vi "isVerbose.vi"(11 "Test Assert in":refnum<class "Test Assert.lvclass">) -> (2 "Verbose":bool, 3 "Test Assert out":refnum<class "Test Assert.lvclass">)   [LabVIEW 2013, in "Caraya.lvlib" / "Test Assert.lvclass"]
uses:
  Test Assert.lvclass
  Test Assert.lvclass/Test Assert.ctl
  Test Manager/Test Manager.lvclass/Test Manager.ctl
  Test Manager/Test Manager.lvclass
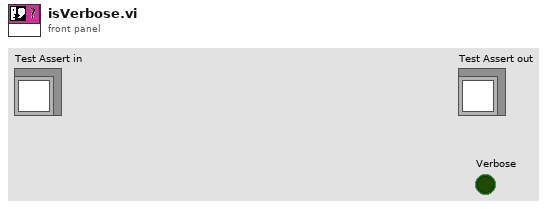
[diagram p1: front panel]
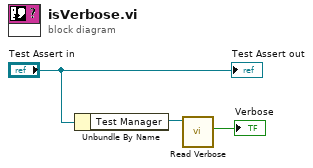
[diagram p0: block diagram]
diagram:
  n1 = Unbundle By Name("Test Assert in") -> ("Test Manager"=w2:refnum<class "Test Manager.lvclass">)
  n2 = call "Read Verbose.vi"("Test Manager"=w2) -> ("Verbose"=→"Verbose":bool)  [unwired: 8 in, 2 out]
  "Test Assert out" <- "Test Assert in"
